vi "Set.vi"(8 "error in (no error)":errorcluster, 9 "status in":T2 items=["Closed", "Open"], 10 "valve in":T1 items=["Valve 1"=1, "Valve 2"=2, "Valve 3"=3, "Valve 4"=4, "Valve 5"=5, "Valve 6"=6, "Valve 7"=7], 11 "INL Valve Controller in":refnum<class "INL Valve Controller.lvclass">) -> (0 "error out":errorcluster, 1 "status out":T2 items=["Closed", "Open"], 2 "Valve out":T1=7 items=["Valve 1"=1, "Valve 2"=2, "Valve 3"=3, "Valve 4"=4, "Valve 5"=5, "Valve 6"=6, "Valve 7"=7], 3 "INL Valve Controller out":refnum<class "INL Valve Controller.lvclass">)   [LabVIEW 2011, in "INL Valve Controller.lvclass"]
uses:
  INL Valve Controller.lvclass
  Valve Controller/Status.ctl
  Valve Controller/Valves.ctl
  INL Valve Controller.lvclass/INL Valve Controller.ctl
  Valve Controller/Valve Controller.lvclass
panel:
  out "read buffer":string
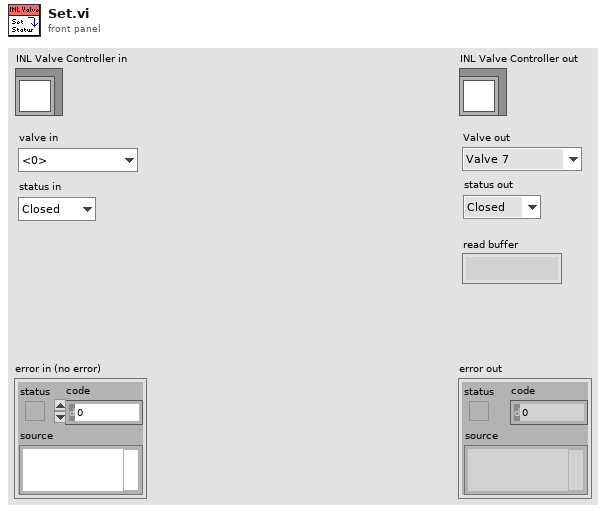
[diagram p1: front panel]
types:
  T1 = typedef "Valve Controller.lvclass/Valves.ctl" = u16
  T2 = typedef "Valve Controller.lvclass/Status.ctl" = u16
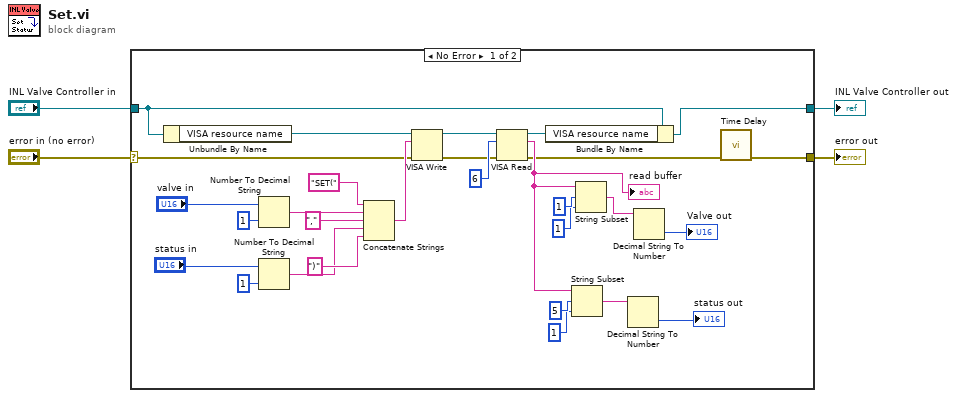
[diagram p0: block diagram]
diagram:
  n1 = case shown="No Error" "error in (no error)" {
    selector: "error in (no error)" -> [w7 w35]
    tunnel: [w6 w35] -> w3
    tunnel: [w5 w34] -> w1
    tunnel: "INL Valve Controller in" -> [w9 w34]
    frame No Error {
      n2 = Unbundle By Name(w9) -> ("VISA resource name"=w8:refnum<visa-resource-name>)
      n3 = Number To Decimal String(number="valve in", width (-)=i16 1) -> (decimal integer string=w13:string)
      n4 = Number To Decimal String(number="status in", width (-)=i16 1) -> (decimal integer string=w15:string)
      n5 = Concatenate Strings("SET(", w13, ",", w15, ")") -> (w18:string)
      n6 = VISA Write(VISA resource name=w8, write buffer=w18, error in (no error)=w7) -> (VISA resource name out=w20:refnum<visa-resource-name>, error out=w19:errorcluster)  [unwired: 1 out]
      n7 = VISA Read(VISA resource name=w20, byte count=u32 6, error in (no error)=w19) -> (VISA resource name out=w21:refnum<visa-resource-name>, read buffer=w30:string, error out=w22:errorcluster)  [unwired: 1 out]
      "read buffer" <- w30
      n8 = Bundle By Name(cluster=w9, "VISA resource name"=w21) -> (w5:refnum<class "INL Valve Controller.lvclass">)
      n9 = String Subset(string=w30, offset (0)=5, length (rest)=1 ("length (rest)")) -> (substring=w29:string)
      n10 = String Subset(string=w30, offset (0)=1, length (rest)=1 ("length (rest)")) -> (substring=w26:string)
      n11 = Decimal String To Number(string=w29) -> (number=→"status out":i32)  [unwired: 2 in, 1 out]
      n12 = Decimal String To Number(string=w26) -> (number=→"Valve out":i32)  [unwired: 2 in, 1 out]
      n13 = call "Time Delay"("error in (no error)"=w22) -> ("error out"=w6:errorcluster)  [unwired: 10 in]
    }
    frame Error {
    }
  }
  "error out" <- w3
  "INL Valve Controller out" <- w1
